vi "Release Address.vi"(10 "Actor":refnum<class "Actor.lvclass">) -> (2 "Unhandled Msgs":refnum<class "Msg.lvclass">[](array[class]))   [LabVIEW 2020, in "jettl.lvlib" / "Actor.lvlib"]
uses:
  Actor.lvlib
  Actor/Actor.lvclass
  Msg/Msg.lvclass
  Attributes/Attributes/Attributes.lvclass
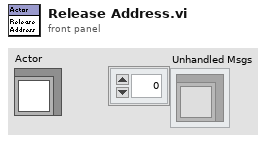
[diagram p1: front panel]
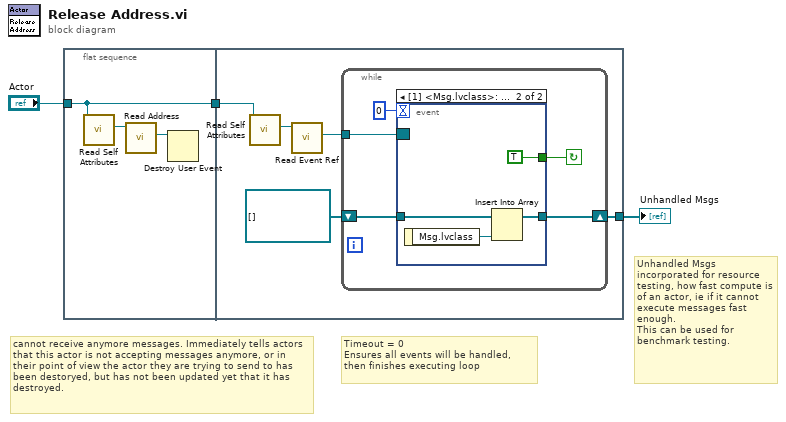
[diagram p0: block diagram]
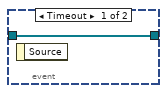
[diagram p2: hidden frame]
diagram:
  # "Unhandled Msgs incorporated for resource testing, how fast compute is of an actor, ie if it cannot execute messages fast enough.\nThis can be used for benchmark testing."
  # "Timeout = 0\nEnsures all events will be handled, then finishes executing loop"
  # "cannot receive anymore messages. Immediately tells actors that this actor is not accepting messages anymore, or in their point of view the actor they are trying to send to has been destoryed, but has not been updated yet that it has destroyed."
  n1 = flat-sequence {
    tunnel: "Actor" -> [w4]
    tunnel: [w4] -> w1
    tunnel: [w7] -> w3
    tunnel: w1 -> [w10]
    frame #0 {
      n2 = call-dynamic "Read Self Attributes.vi"("Actor in"=w4) -> ("Self Attributes"=w6:refnum<class "Attributes.lvclass">)  [unwired: 10 in]
      n3 = call-dynamic "Read Address.vi"("Attributes in"=w6) -> ("Address"=w5:refnum<user-event>)  [unwired: 10 in]
      n4 = Destroy User Event(user event=w5) -> ()  [unwired: 1 in, 1 out]
    }
    frame #1 {
      n5 = call-dynamic "Read Self Attributes.vi"("Actor in"=w10) -> ("Self Attributes"=w11:refnum<class "Attributes.lvclass">)  [unwired: 10 in]
      n6 = call-dynamic "Read Event Ref.vi"("Attributes in"=w11) -> ("Event Ref"=w8:refnum<event-registration>)  [unwired: 10 in]
      n7 = while {
        shift-right: [w15] -> w7
        shift-left: refnum<class "Msg.lvclass">[] [] -> [w16]
        tunnel: w8 -> [w14]
        stop <- w13 continue-if-true
        n8 = event shown="[1] <Msg.lvclass>: User Event" {
          selector: w14 -> [_ _]
          dyn-events: _ -> [_ _]
          timeout: 0 -> [_ _]
          tunnel: w16 -> [w17 w21]
          tunnel: [w17 w20] -> w15
          tunnel: [_ TRUE] -> w13
          event Timeout {
            n9 = event-data() -> ()  [unwired: 1 in, 1 out]
          }
          event User Event {
            n10 = event-data() -> ("Msg.lvclass"=w19:refnum<class "Msg.lvclass">)  [unwired: 1 in]
            n11 = Insert Into Array(array=w21, new element=w19) -> (w20:refnum<class "Msg.lvclass">[])  [unwired: 1 in]
          }
        }
      }
    }
  }
  "Unhandled Msgs" <- w3
